vi "WPI_AnalogModuleGetAverageVoltage.vi"(8 "error in (no error)":errorcluster, 10 "Channel":T2=enum."AI 1", 11 "AnalogModuleDevStatus":T1) -> (0 "error out":errorcluster, 2 "Average Voltage":dbl, 3 "AnalogModuleDevStatus":T1)   [LabVIEW 2017]
doc: "This software is licensed. Open the labview\\readme\\WPI Robotics Library Open Source License.txt file for more information."
uses:
  <vilib>/Rock Robotics/SystemInterfaces/AI/FPGA_AIChannel.ctl
  <vilib>/Rock Robotics/WPI/AnalogModule/WPI_AnalogModuleDevStatus.ctl
  <vilib>/Rock Robotics/SystemInterfaces/System/FPGA_SystemGet.vi
  <vilib>/Rock Robotics/SystemInterfaces/AI/FPGA_AIOversampleBits.vi
  <vilib>/Rock Robotics/SystemInterfaces/AI/FPGA_AIERRInvalidAnalogChannel.vi
  <vilib>/Rock Robotics/SystemInterfaces/AI/FPGA_ReadAI.vi
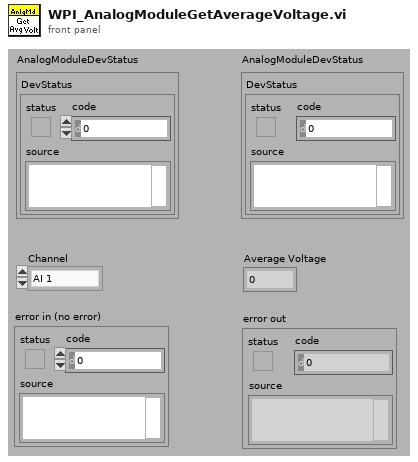
[diagram p1: front panel]
types:
  T1 = typedef "WPI_AnalogModuleDevStatus.ctl" = cluster{"DevStatus":errorcluster}
  T2 = typedef "FPGA_AIChannel.ctl" = enum8{"AI 0", "AI 1", "AI 2", "AI 3", "AI MXP 0", "AI MXP 1", "AI MXP 2", "AI MXP 3", "Invalid"}
  T3 = typedef "FPGA_AIDevRef.ctl" = cluster{"DevStatus":errorcluster}
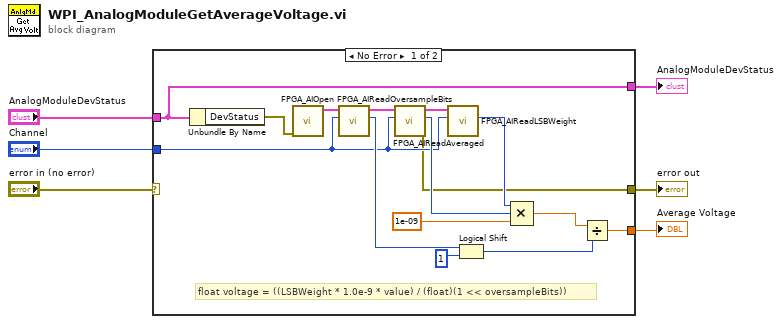
[diagram p0: block diagram]
diagram:
  n1 = case shown="No Error" "error in (no error)" {
    selector: "error in (no error)" -> [_ w23]
    tunnel: "AnalogModuleDevStatus" -> [w10 w22]
    tunnel: [w10 w22] -> w5
    tunnel: "Channel" -> [w13 _]
    tunnel: [w8 _] -> w3
    tunnel: [w9 w23] -> w1
    frame No Error {
      # "float voltage = ((LSBWeight * 1.0e-9 * value) / (float)(1 << oversampleBits))"
      n2 = Unbundle By Name(w10) -> ("DevStatus"=w21:errorcluster)
      n3 = call <vilib>:"FPGA_AIOpen.vi"("error in (no error)"=w21) -> ("AI Reference out"=w12:T3)  [unwired: 2 in, 8 out]
      n4 = call <vilib>:"FPGA_AIReadOversampleBits.vi"("Channel"=w13, "AI Reference in"=w12) -> ("OversampleBits"=w14:u8, "AI Reference out"=w11:T3)  [unwired: 2 in, 6 out]
      n5 = call <vilib>:"FPGA_AIReadAveraged.vi"("Channel"=w13, "AI Reference in"=w11) -> ("error out"=w9:errorcluster, "Averaged"=w17:i32, "AI Reference out"=w19:T3)  [unwired: 1 in, 6 out]
      n6 = call <vilib>:"FPGA_AIReadLSBWeight.vi"("Channel"=w13, "AI Reference"=w19) -> ("LSBWeight"=w18:u32)  [unwired: 1 in, 8 out]
      n7 = Logical Shift(y=w14, x=u32 1) -> (x << y=w7:u32)
      n8 = Compound Arithmetic op=MULTIPLY(w18, w17, 1e-09 ("y")) -> (w15:dbl)
      n9 = Divide(x=w15, y=w7) -> (x/y=w8:dbl)
    }
    frame Error {
    }
  }
  "AnalogModuleDevStatus" <- w5
  "Average Voltage" <- w3
  "error out" <- w1
